vi "Easy Parse XML.vi"(8 "error in (no error)":errorcluster, 9 "LabVIEW Data (Type)":variant, 10 "XML String":string) -> (0 "error out":errorcluster, 2 "LabVIEW Data":variant)   [LabVIEW 2011]
doc: "Converts an <B>XML String</B> to <B>LabVIEW Data</B>, based on the <B>LabVIEW Data (Type)</B> argument. Use the <B>Variant to Data</B> function to convert the output variant <B>LabVIEW Data</B> to the desired data type."
panel:
  # "JKI EasyXML Toolkit for LabVIEW\nhttp://jki.net/easyxml\nCopyright (C) 2007-2015, JKI <info@jki.net>\nALL RIGHTS RESERVED"
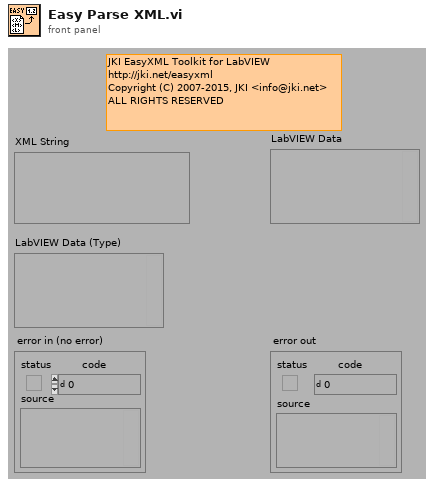
[diagram p1: front panel]
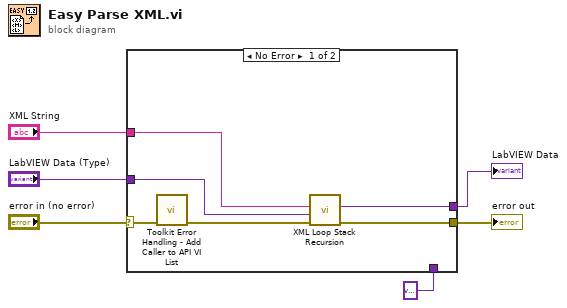
[diagram p0: block diagram]
diagram:
  n1 = case shown="No Error" "error in (no error)" {
    selector: "error in (no error)" -> [w12 w14]
    tunnel: [w7 w14] -> w5
    tunnel: "LabVIEW Data (Type)" -> [w11 _]
    tunnel: variant ("LabVIEW Data") -> [_ w13]
    tunnel: "XML String" -> [w9 _]
    tunnel: [w10 w13] -> w2
    frame No Error {
      n2 = call "Toolkit Error Handling - Add Caller to API VI List.vi"("error in"=w12) -> ("error out"=w8:errorcluster)  [unwired: 10 in]
      n3 = call "XML Loop Stack Recursion.vi"("error in"=w8, "type"=w11, "xml string"=w9) -> ("error out"=w7:errorcluster, "data out"=w10:variant)  [unwired: 7 in]
    }
    frame Error {
    }
  }
  "error out" <- w5
  "LabVIEW Data" <- w2
